vi "Destructor.vi"(8 "error in":errorcluster, 11 "CustomElement":refnum<class "CustomElement.lvclass">) -> (0 "error out":errorcluster)   [LabVIEW 2021, in "ProligentXMLGenerator.lvlib" / "CustomElement.lvclass"]
uses:
  CustomElement.lvclass
  CustomElement.lvclass/CustomElement.ctl
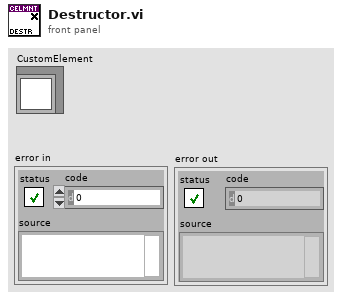
[diagram p1: front panel]
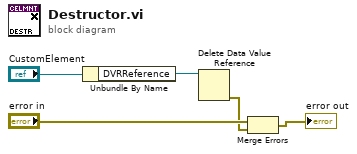
[diagram p0: block diagram]
diagram:
  n1 = Unbundle By Name("CustomElement") -> ("DVRReference"=w2:refnum<data-value>)
  n2 = Delete Data Value Reference(data value reference=w2) -> (error out=w3:errorcluster)  [unwired: 1 in, 1 out]
  n3 = Merge Errors("error in", w3) -> (→"error out":errorcluster)
